vi "Import.vi"(6 "Import Mode":u32(ring) items=["merge"=0, "replace all"=1048576, "preserve existing"=2097152], 8 "error in (no error)":errorcluster, 9 "Experts":string, 10 "Source File":path, 11 "Session in":refnum<k21>="localhost") -> (0 "error out":errorcluster, 2 "Detailed Result":string, 3 "Session out":refnum<k21>)   [LabVIEW 2020, in "nisyscfg.lvlib"]
doc: "Use this VI to import configuration data from a file into MAX. Not all products are supported; consult your product documentation."
uses:
  <vilib>/nisyscfg/nisyscfg.lvlib
  <vilib>/Utility/error.llb/Error Cluster From Error Code.vi
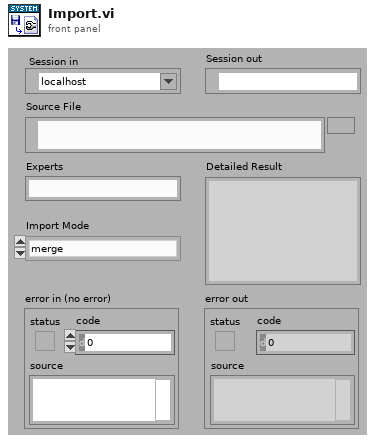
[diagram p1: front panel]
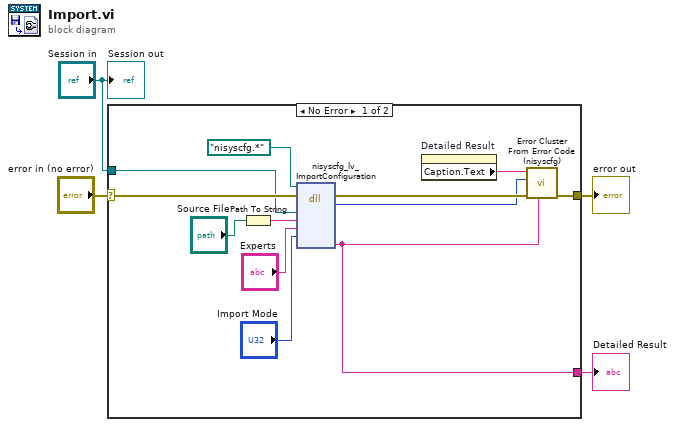
[diagram p0: block diagram]
diagram:
  n1 = case shown="No Error" "error in (no error)" {
    selector: "error in (no error)" -> [w12 w17]
    tunnel: [w8 w17] -> w4
    tunnel: "Session in" -> [w11 _]
    tunnel: [w7 _] -> w1
    frame No Error {
      n2 = Path To String(path="Source File") -> (string=w15:string)
      n3 = dll-call lib="nisyscfg.*" fn="nisyscfg_lv_ImportConfiguration" label="ImportConfiguration"(path in=path "nisyscfg.*", error in=w12, "sessionHandle"=w11, "sourceFilename"=w15, "expertNames"="Experts", "importMode"="Import Mode") -> (error out=w9:errorcluster, "return type"=w5:i32, "detailedResult"=w7:string)  [unwired: 6 in, 1 out]
      n4 = property on="Detailed Result" class="Str"() -> ("Caption.Text"=w6:string)  [unwired: 2 in, 2 out]
      n5 = call <vilib>:"Error Cluster From Error Code (nisyscfg).vi"("Details String"=w7, "error in (no error)"=w9, "Error Code (0)"=w5, "Details Caption"=w6) -> ("error out"=w8:errorcluster)  [unwired: 7 in]
    }
    frame Error {
    }
  }
  "error out" <- w4
  "Detailed Result" <- w1
  "Session out" <- "Session in"
